vi "stateMain.vi"() -> ()   [LabVIEW 2012]
doc: "Use this template to build a simple state machine design pattern. Each state executes code and determines which state to transition to."
uses:
  controls/stateState.ctl
  controls/stateData.ctl
panel:
  in  "Do Something Else <Replace Me>":bool
  in  "Do Something <Replace Me>":bool
  in  "Stop Button":bool
  # "These controls have associated \"Value Changed\" events configured in the Event Structure on the diagram.\n\nReplace them (and reconfigure the Event Structure) with the controls you need for your application."
  # "This template is for the Simple State Machine design pattern.\n\nSee the block diagram for more information on how to use this template."
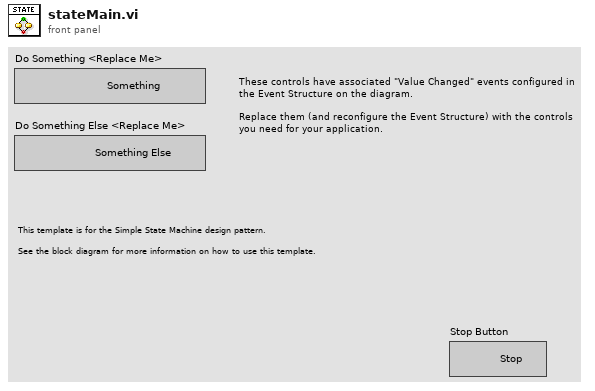
[diagram p1: front panel]
types:
  T1 = typedef "stateData.ctl" = cluster{"Boolean <Replace Me>":bool, "String <Replace Me>":string, "Numeric <Replace Me>":dbl}
  T2 = typedef "stateState.ctl" = enum16{"Initialize", "Wait for Event", "User State 1", "User State 2", "Stop"}
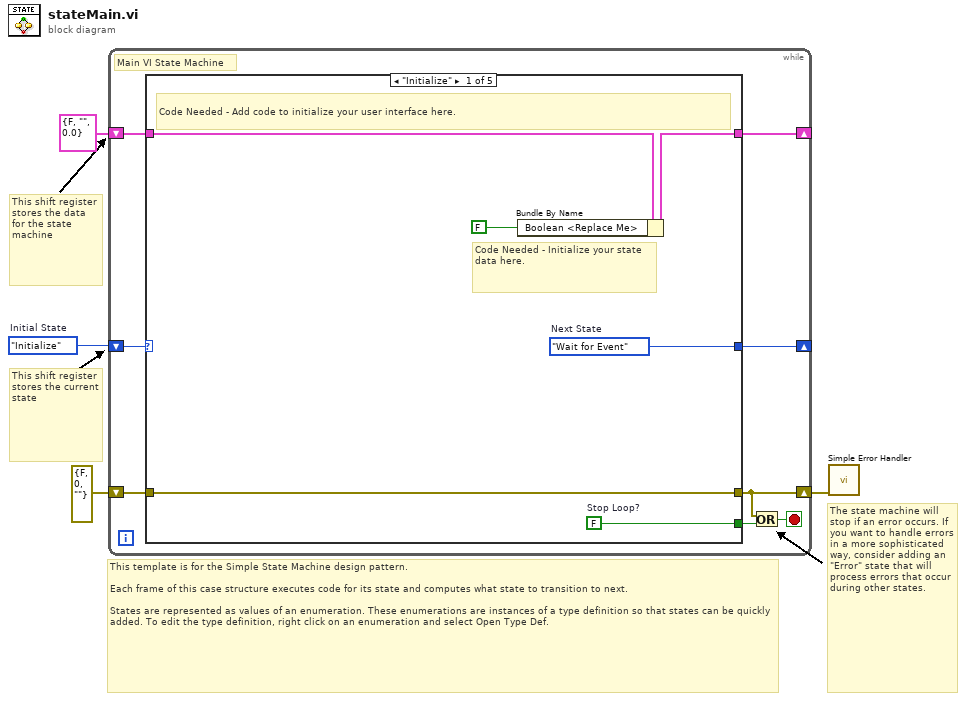
[diagram p0: block diagram]
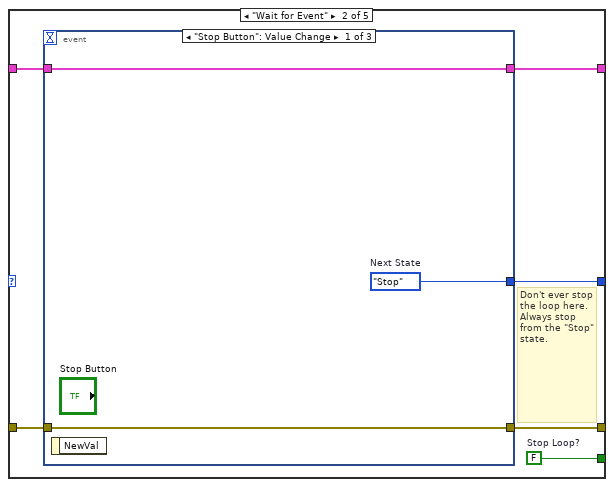
[diagram p2: hidden frame]
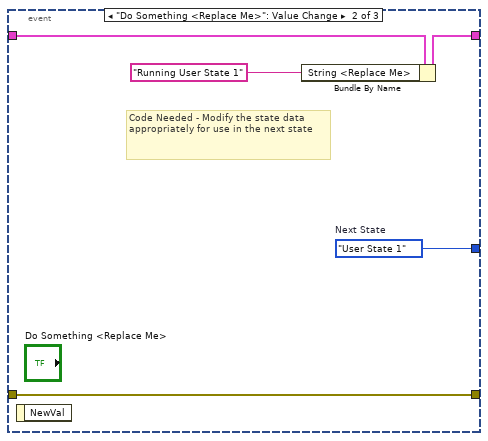
[diagram p3: hidden frame]
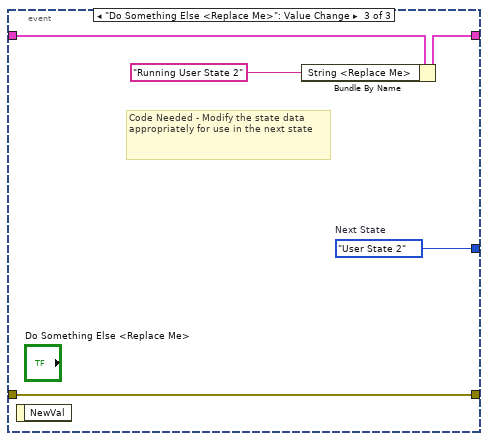
[diagram p4: hidden frame]
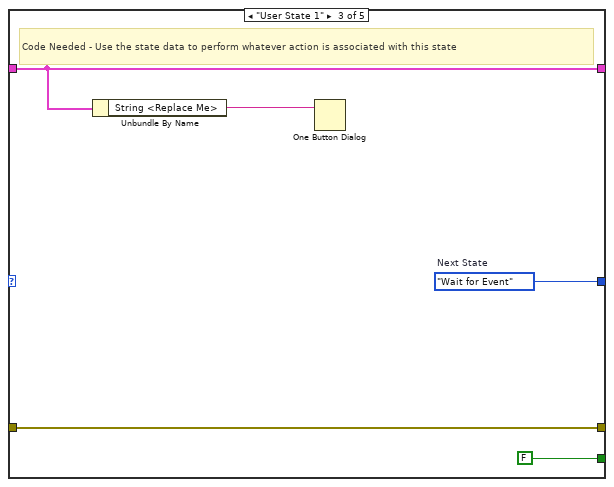
[diagram p5: hidden frame]
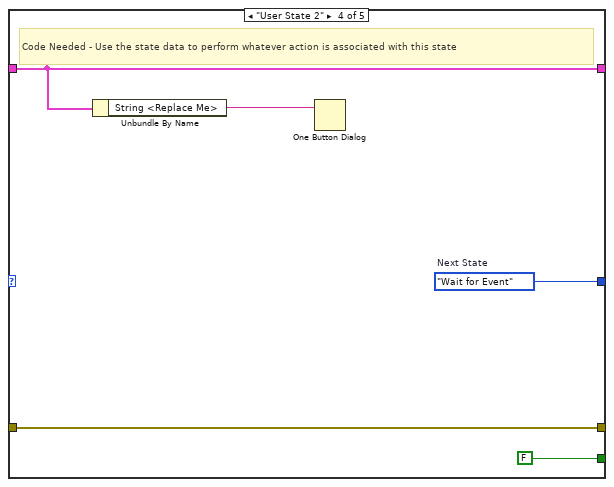
[diagram p6: hidden frame]
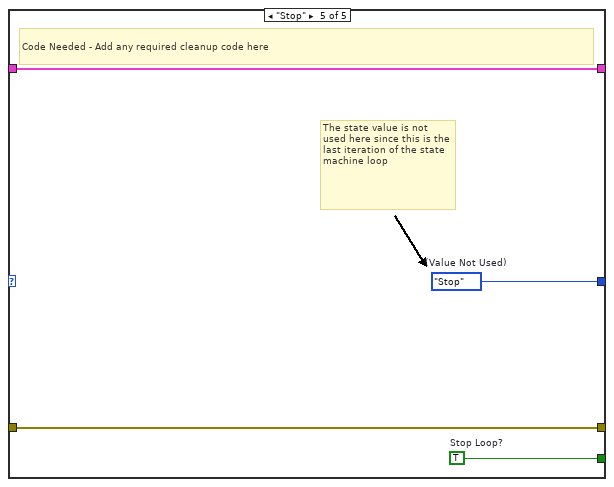
[diagram p7: hidden frame]
diagram:
  w4 = stateState."Initialize"  # Initial State
  # "The state machine will stop if an error occurs. If you want to handle errors in a more sophisticated way, consider adding an \"Error\" state that will process errors that occur during other states."
  # "This shift register\nstores the data for the state machine"
  # "This template is for the Simple State Machine design pattern.\n\nEach frame of this case structure executes code for its state and computes what state to transition to next.\n\nStates are represented as values of an enumeration. These enumerations are instances of a type definition so that states can be quickly added. To edit the type definition, right click on an enumeration and select Open Type Def."
  # "This shift register\nstores the current\nstate"
  n1 = while {
    shift-right: [w11] -> _
    shift-left: w4 -> [w12]
    shift-right: [w9] -> _
    shift-left: T1 {"Boolean <Replace Me>"=FALSE, "String <Replace Me>"="", "Numeric <Replace Me>"=0.0} ("Data") -> [w10]
    shift-right: [w5] -> w1
    shift-left: errorcluster {"status"=FALSE, "code"=0, "source"=""} ("error constant") -> [w8]
    stop <- w6 stop-if-true
    # "Main VI State Machine"
    n2 = case shown="\"Initialize\"" w12 {
      tunnel: [w18 w24 w42 w47 w51] -> w11
      tunnel: [w17 w23 FALSE ("Stop Loop?") FALSE ("Stop Loop?") w49] -> w7
      tunnel: w10 -> [w16 w22 w40 w45 w50]
      tunnel: [w15 w21 w40 w45 w50] -> w9
      tunnel: w8 -> [w13 w20 w38 w43 w48]
      tunnel: [w13 w19 w38 w43 w48] -> w5
      frame "Initialize" {
        w17 = FALSE  # Stop Loop?
        w18 = stateState."Wait for Event"  # Next State
        # "Code Needed - Initialize your state data here."
        # "Code Needed - Add code to initialize your user interface here."
        n3 = Bundle By Name(cluster=w16, "Boolean <Replace Me>"=FALSE ("Replace_Me_Boolean")) -> (w15:T1)
      }
      frame "Wait for Event" {
        w23 = FALSE  # Stop Loop?
        # "Don't ever stop the loop here. Always stop from the \"Stop\" state."
        n4 = event shown="[0] \"Stop Button\": Value Change" {
          selector: _ -> [_ _ _]
          dyn-events: _ -> [_ _ _]
          timeout: _ -> [_ _ _]
          tunnel: [w27 w32 w37] -> w24
          tunnel: w22 -> [w26 w31 w36]
          tunnel: [w26 w30 w35] -> w21
          tunnel: w20 -> [w25 w28 w33]
          tunnel: [w25 w28 w33] -> w19
          event "Stop Button": Value Change {
            w27 = stateState."Stop"  # Next State
            n5 = event-data() -> ()  [unwired: 1 in, 1 out]
          }
          event "Do Something <Replace Me>": Value Change {
            w32 = stateState."User State 1"  # Next State
            # "Code Needed - Modify the state data appropriately for use in the next state"
            n6 = event-data() -> ()  [unwired: 1 in, 1 out]
            n7 = Bundle By Name(cluster=w31, "String <Replace Me>"="Running User State 1" ("Running User State 1")) -> (w30:T1)
          }
          event "Do Something Else <Replace Me>": Value Change {
            w37 = stateState."User State 2"  # Next State
            # "Code Needed - Modify the state data appropriately for use in the next state"
            n8 = event-data() -> ()  [unwired: 1 in, 1 out]
            n9 = Bundle By Name(cluster=w36, "String <Replace Me>"="Running User State 2" ("Running User State 2")) -> (w35:T1)
          }
        }
      }
      frame "User State 1" {
        w42 = stateState."Wait for Event"  # Next State
        # "Code Needed - Use the state data to perform whatever action is associated with this state"
        n10 = Unbundle By Name(w40) -> ("String <Replace Me>"=w39:string)
        n11 = One Button Dialog(message=w39) -> ()  [unwired: 1 in, 1 out]
      }
      frame "User State 2" {
        w47 = stateState."Wait for Event"  # Next State
        # "Code Needed - Use the state data to perform whatever action is associated with this state"
        n12 = Unbundle By Name(w45) -> ("String <Replace Me>"=w44:string)
        n13 = One Button Dialog(message=w44) -> ()  [unwired: 1 in, 1 out]
      }
      frame "Stop" {
        w49 = TRUE  # Stop Loop?
        w51 = stateState."Stop"  # (Value Not Used)
        # "Code Needed - Add any required cleanup code here"
        # "The state value is not used here since this is the last iteration of the state machine loop"
      }
    }
    n14 = Or(x=w5, y=w7) -> (x .or. y?=w6:bool)
  }
  n15 = call <vilib>:"Simple Error Handler.vi"("error in (no error)"=w1) -> ()  [unwired: 4 in, 5 out]
